vi "TematyDane.vi"(9 "Value":u16, 10 "TematyDane in":string[][](array[string]), 11 "Tematy-Lista":string[](array[string])) -> (0 "Array":i32[](array[numeric]), 1 "Dane":string[](array[string]), 2 "Podtemat":string, 3 "Temat":string)   [LabVIEW 2017]
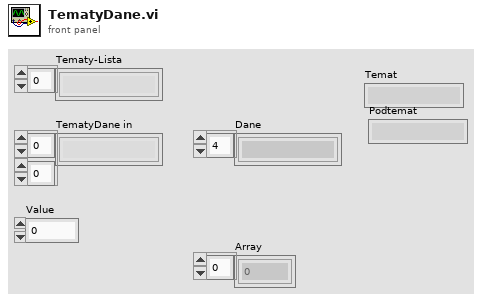
[diagram p1: front panel]
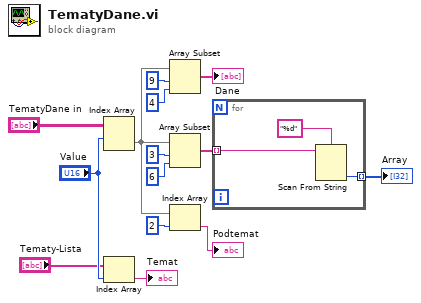
[diagram p0: block diagram]
diagram:
  n1 = Index Array(array="TematyDane in", index (row)="Value") -> (element=w3:string[])  [unwired: 1 in]
  n2 = Index Array(array="Tematy-Lista", index="Value") -> (element=→"Temat":string)
  n3 = Array Subset(array=w3, index=9, length=4) -> (→"Dane":string[])
  n4 = Array Subset(array=w3, index=3, length=6) -> (w10:string[])
  n5 = Index Array(array=w3, index=2) -> (element=→"Podtemat":string)
  n6 = for {
    tunnel: w10 -> [w17] mode=indexing
    tunnel: [w16] -> w11 mode=indexing
    n7 = Scan From String(format string="%d", input string=w17) -> (output 1=w16:i32)  [unwired: 3 in, 3 out]
  }
  "Array" <- w11
